vi "MPS_transmit_receive.vi"(4 "samples per readout":i32=16000, 5 "Use Bias?":bool, 9 "InputChans":enum16{"Rx", "BiasIMon", "TxIMon", "BMon"}(ring), 10 "channel input for max readouts":T1, 11 "Measurement Queue":refnum<queue>) -> ()   [LabVIEW 2021]
doc: "This VI is responsible for collecting the data of the MPI experiment from the DAQ and it writes the data of the output waveforms to the DAQ. Generally, this VI can be operated in two modes: Continuous or non-continuous mode. In non-continuous mode, a finite number of samples is read from the ADC and a finite number of samples is written to the DAC. After playing these waveforms and acquiring the samples, the VI stops. The number of samples is determined by the product of \"samples per readout\" and the \"max readouts\" number passed to the VI via a channel structure. The latter allows to update the stopping condition while the acquisition is already running. Acquired data is written to a queue (has to be provided as an input) from which the main VI can then dequeue the readout buckets. Therefore, the sub-VI can be seen as the producer loop while the consumer loop is located in the main VI.\nIn continuous mode, a finite waveform sample is repeated over and over until the data acquisition reaches the set limit or it is stopped. \nInternally, the VI has three different DAQ tasks: Analog input acquisition, analog output generation and digital input acquisition. The analog input acquisition task is the \"master task\" and all other tasks are triggered when the analog data acquisition starts. \nMost of the DAQ settings are read from the global variables (including channel, channel type and sampling rate).\nThe rotary position is taken in the middle of the readout bucket. \nFor safety reasons, the VI ensures that zeros are written to the DAQ when stopping the VI properly."
uses:
  <extravilib>/ChannelInstances/Tag-dbl/))Channel.ctl
  <vilib>/DAQmx/write.llb/DAQmx Write (Analog 1D Wfm NChan NSamp).vi
  <vilib>/DAQmx/read.llb/DAQmx Read (Analog Wfm 1Chan NSamp).vi
  MPS_global_variables.vi
  <vilib>/DAQmx/create/channels.llb/DAQmx Create Channel (AI-Voltage-Basic).vi
  <vilib>/DAQmx/configure/timing.llb/DAQmx Timing (Sample Clock).vi
  <vilib>/DAQmx/configure/trigger.llb/DAQmx Start Trigger (None).vi
  <vilib>/Waveform/WDTOps.llb/WDT Number of Waveform Samples DBL.vi
  <vilib>/DAQmx/create/channels.llb/DAQmx Create Channel (AO-Voltage-Basic).vi
  <vilib>/DAQmx/configure/trigger.llb/DAQmx Start Trigger (Digital Edge).vi
  <vilib>/DAQmx/miscellaneous.llb/DAQmx Fill In Error Info.vi
  <extravilib>/ChannelInstances/Tag-dbl/EndpointRead.vi
  <extravilib>/ChannelInstances/Tag-dbl.lvlib
  <resource>/objmgr/daqmx.rc
  <vilib>/measure/NI_MABase.lvlib
panel:
  out "output cluster":cluster{"Fs":dbl, "#s":dbl}
  out "Input waveforms 2":dbl[](graph)
  out "sample rate":dbl
  out "Sample rate actual":dbl
  out "number of samples written per channel":u32
  out "AI while loop i":i32
  out "AO while loop i":i32
  out "element":dbl
  out "Input waveforms":dynamicdata(graph)=[{"t0"=timestamp(5.936 s since 1904-01-01), "dt"=1e-06, "Y"=array[16000 elements]}, {"t0"=timestamp(5.936 s since 1904-01-01), "dt"=1e-06, "Y"=array[16000 elements]}]
  out "Transmit stopped":bool=TRUE
  out "current readout no":i32
  out "RX":waveform(dbl)(graph)
  out "Data aquisition stopped":bool=TRUE
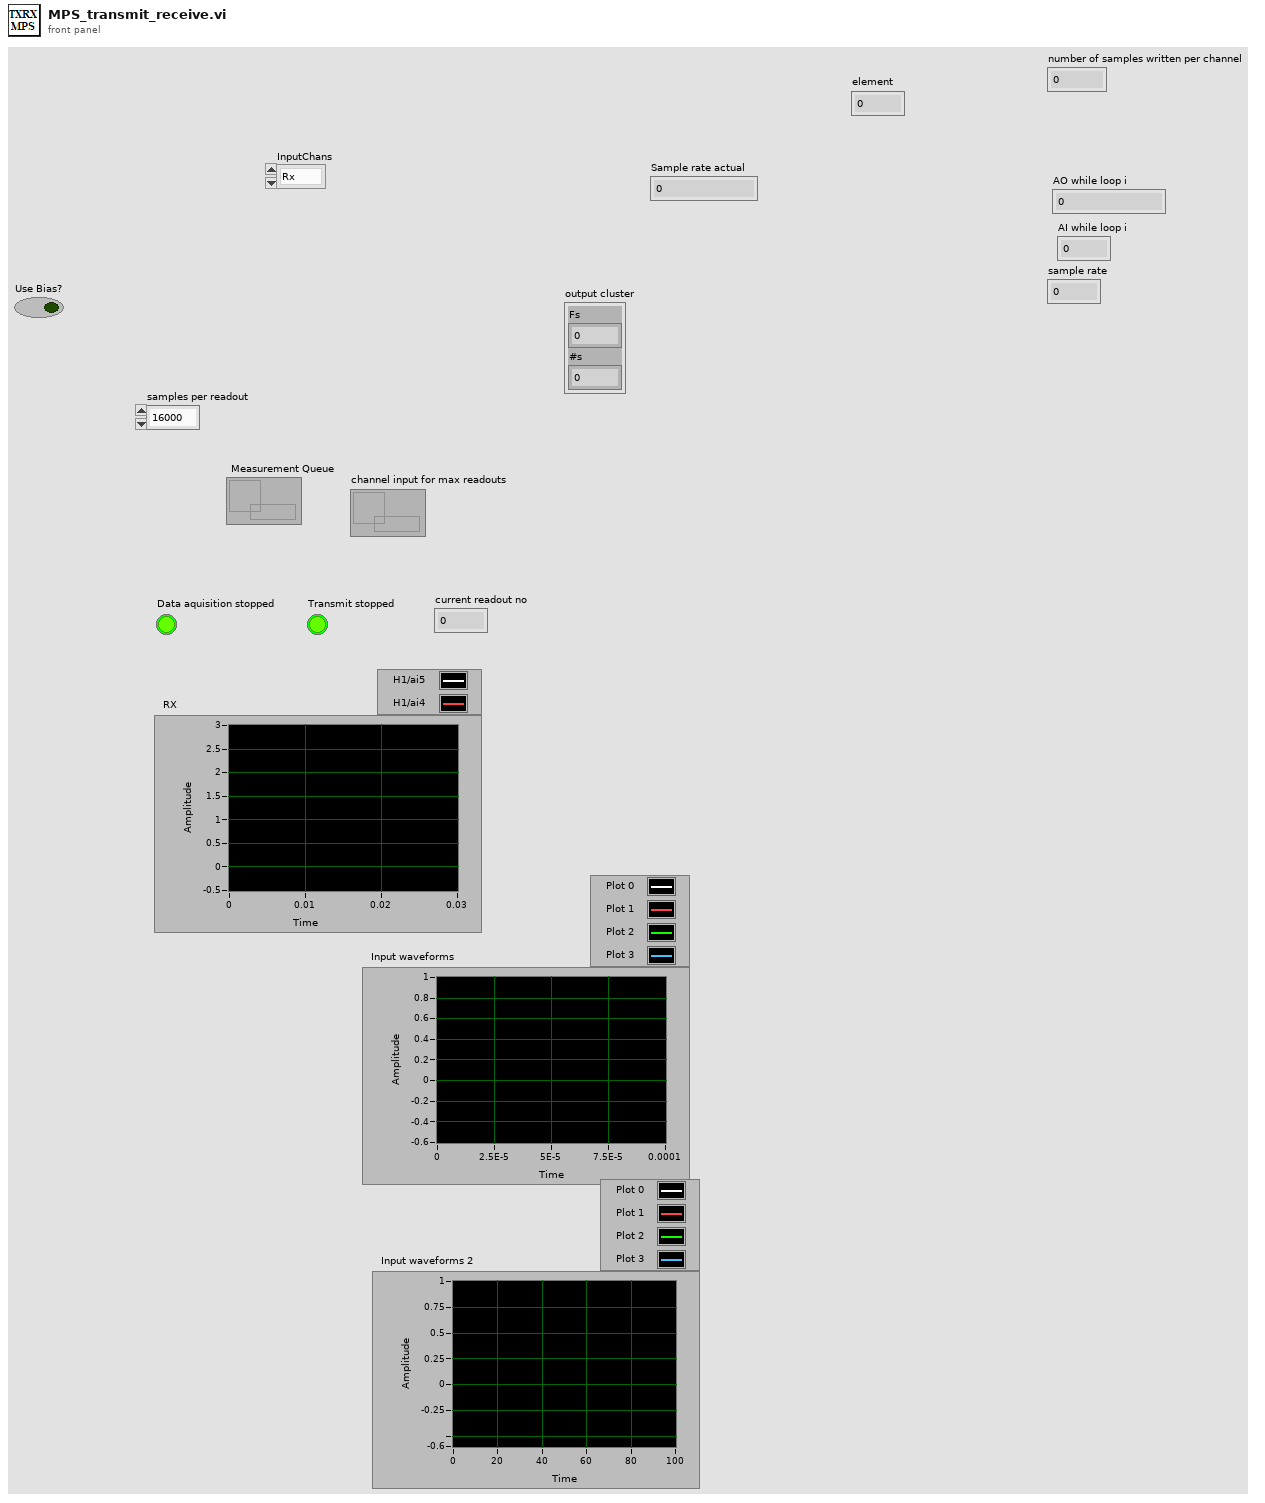
[diagram p1: front panel]
types:
  T1 = typedef "Tag-dbl.lvlib/))Channel.ctl" = refnum<queue>
  T2 = cluster{"sample rate":dbl, "Tx freq":dbl, "Tx amp":dbl, "Tx cycles\nSpectroscopy":dbl, "Bias amp":dbl, "Bias freq":dbl, "Receive range":dbl, "Bias Periods\nMagnetometry":dbl, "Tx Freq Division Factor":dbl, "Drive Periods per Bias":dbl, "TX harmonics":dbl[]}
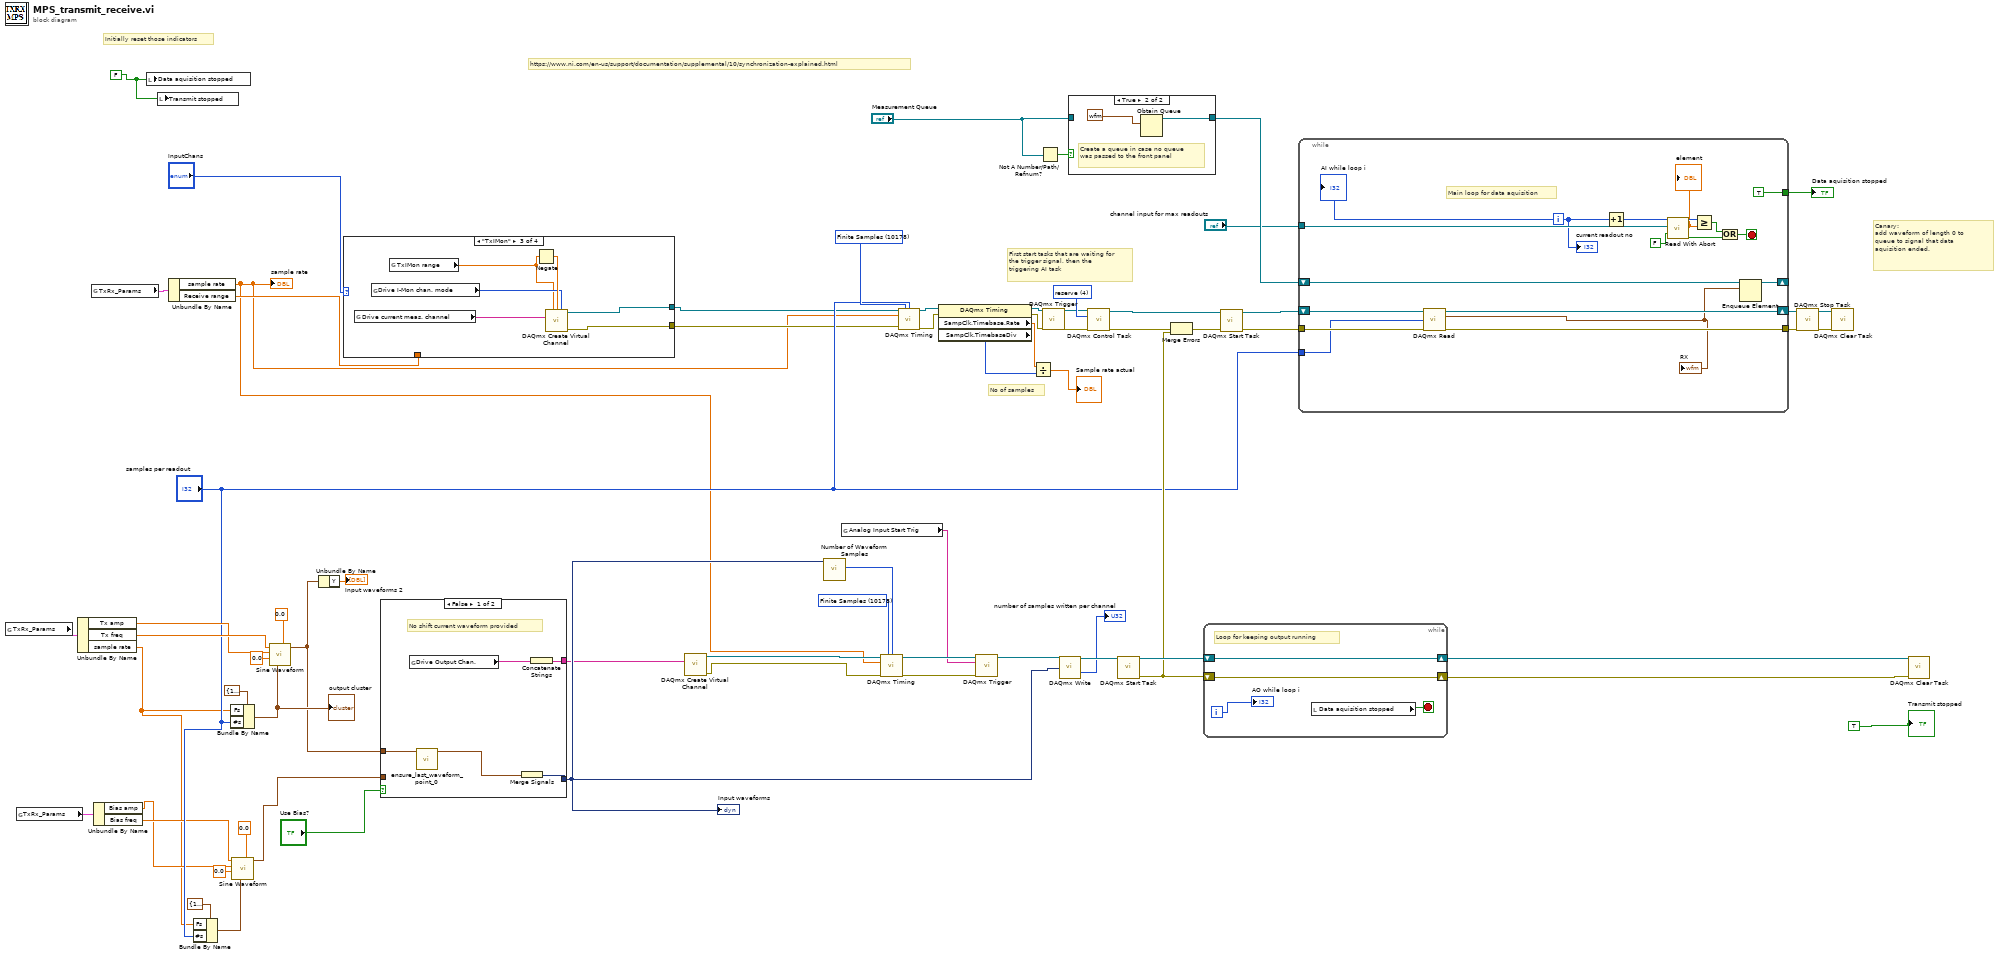
[diagram p0: block diagram]
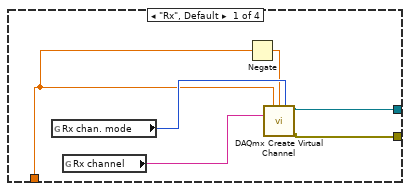
[diagram p2: hidden frame]
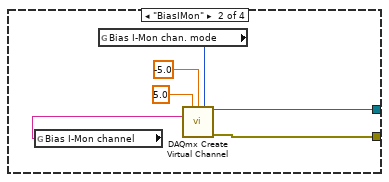
[diagram p3: hidden frame]
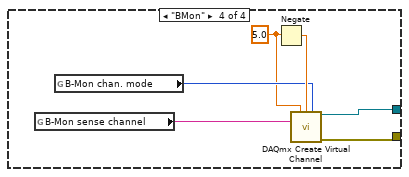
[diagram p4: hidden frame]
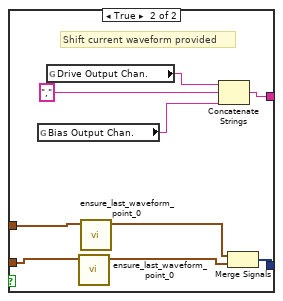
[diagram p6: hidden frame]
diagram:
  w47 = 10178 items=["Finite Samples"=10178, "Continuous Samples"=10123, "Hardware Timed Single Point"=12522] ("sample mode")
  w56 = 4 items=["verify"=2, "reserve"=4, "commit"=3, "unreserve"=5, "abort"=6] ("action")
  w31 = 10178 items=["Finite Samples"=10178, "Continuous Samples"=10123, "Hardware Timed Single Point"=12522] ("sample mode")
  w52 = FALSE ("Data aquisition stopped 2")
  # "https://www.ni.com/en-us/support/documentation/supplemental/10/synchronization-explained.html"
  # "First start tasks that are waiting for the trigger signal, then the triggering AI task"
  # "Initially reset those indicators"
  # "Canary:\nadd waveform of length 0 to queue to signal that data aquisition ended."
  # "No of samples"
  n1 = global read "MPS_global_variables.vi" "TxRx_Params"() -> (w27:T2)
  n2 = global read "MPS_global_variables.vi" "TxRx_Params"() -> (w26:T2)
  n3 = Unbundle By Name(w27) -> ("Tx amp"=w19:dbl, "Tx freq"=w20:dbl, "sample rate"=w11:dbl)
  n4 = global read "MPS_global_variables.vi" "TxRx_Params"() -> (w33:T2)
  n5 = Unbundle By Name(w26) -> ("Bias amp"=w12:dbl, "Bias freq"=w13:dbl)
  n6 = local write "Data aquisition stopped"(w52) -> ()
  n7 = local write "Transmit stopped"(w52) -> ()
  n8 = Unbundle By Name(w33) -> ("sample rate"=w1:dbl, "Receive range"=w5:dbl)
  "sample rate" <- w1
  n9 = Bundle By Name(cluster=cluster{"Fs":dbl, "#s":dbl} {"Fs"=1000.0, "#s"=1000.0} ("sampling info"), "Fs"=w11, "#s"="samples per readout") -> (w18:cluster{"Fs":dbl, "#s":dbl})
  n10 = Bundle By Name(cluster=cluster{"Fs":dbl, "#s":dbl} {"Fs"=1000.0, "#s"=1000.0} ("sampling info"), "Fs"=w11, "#s"="samples per readout") -> (w21:cluster{"Fs":dbl, "#s":dbl})
  "output cluster" <- w21
  n11 = call <vilib>:"Sine Waveform.vi"("offset"=0.0, "sampling info"=w18, "phase"=0.0, "amplitude"=w12, "frequency"=w13) -> ("signal out"=w14:waveform(dbl))  [unwired: 5 in, 1 out]
  n12 = call <vilib>:"Sine Waveform.vi"("offset"=0.0, "sampling info"=w21, "phase"=0.0, "amplitude"=w19, "frequency"=w20) -> ("signal out"=w8:waveform(dbl))  [unwired: 5 in, 1 out]
  n13 = Unbundle By Name(w8) -> ("Y"=→"Input waveforms 2":dbl[])
  n14 = case shown="\"TxIMon\"" "InputChans" {
    tunnel: w5 -> [w72 _ _ _]
    tunnel: [w71 w77 w84 w89] -> w4
    tunnel: [w70 w76 w83 w88] -> w3
    frame "Rx", Default {
      n15 = global read "MPS_global_variables.vi" "Rx chan. mode"() -> (w74:i32)
      n16 = global read "MPS_global_variables.vi" "Rx channel"() -> (w75:tag)
      n17 = Negate(x=w72) -> (-x=w73:dbl)
      n18 = call-poly <vilib>:"DAQmx Create Virtual Channel.vi"("maximum value"=w72, "minimum value"=w73, "input terminal configuration"=w74, "physical channels"=w75) -> ("task out"=w71:refnum<k21>, "error out"=w70:errorcluster)  [unwired: 10 in]
    }
    frame "BiasIMon" {
      n19 = global read "MPS_global_variables.vi" "Bias I-Mon channel"() -> (w79:tag)
      n20 = global read "MPS_global_variables.vi" "Bias I-Mon chan. mode"() -> (w78:i32)
      n21 = call-poly <vilib>:"DAQmx Create Virtual Channel.vi"("maximum value"=5.0, "minimum value"=-5.0, "input terminal configuration"=w78, "physical channels"=w79) -> ("task out"=w77:refnum<k21>, "error out"=w76:errorcluster)  [unwired: 10 in]
    }
    frame "TxIMon" {
      n22 = global read "MPS_global_variables.vi" "Drive current meas. channel"() -> (w86:tag)
      n23 = global read "MPS_global_variables.vi" "Drive I-Mon chan. mode"() -> (w85:i32)
      n24 = global read "MPS_global_variables.vi" "TxIMon range"() -> (w82:dbl)
      n25 = Negate(x=w82) -> (-x=w87:dbl)
      n26 = call-poly <vilib>:"DAQmx Create Virtual Channel.vi"("maximum value"=w82, "minimum value"=w87, "input terminal configuration"=w85, "physical channels"=w86) -> ("task out"=w84:refnum<k21>, "error out"=w83:errorcluster)  [unwired: 10 in]
    }
    frame "BMon" {
      w90 = 5.0 ("Receive range")
      n27 = global read "MPS_global_variables.vi" "B-Mon sense channel"() -> (w92:tag)
      n28 = global read "MPS_global_variables.vi" "B-Mon chan. mode"() -> (w91:i32)
      n29 = Negate(x=w90) -> (-x=w93:dbl)
      n30 = call-poly <vilib>:"DAQmx Create Virtual Channel.vi"("maximum value"=w90, "minimum value"=w93, "input terminal configuration"=w91, "physical channels"=w92) -> ("task out"=w89:refnum<k21>, "error out"=w88:errorcluster)  [unwired: 10 in]
    }
  }
  n31 = case shown="False" "Use Bias?" {
    tunnel: [w96 w107] -> w32
    tunnel: w14 -> [_ w104]
    tunnel: w8 -> [w97 w101]
    tunnel: [w98 w106] -> w59
    frame False {
      # "No shift current waveform provided"
      n32 = global read "MPS_global_variables.vi" "Drive Output Chan."() -> (w94:tag)
      n33 = call "ensure_last_waveform_point_0.vi"("Waveform in"=w97) -> ("Waveform out"=w95:waveform(dbl))  [unwired: 10 in]
      n34 = Merge Signals(w95) -> (w98:dynamicdata)
      n35 = Concatenate Strings(w94) -> (w96:string)
    }
    frame True {
      # "Shift current waveform provided"
      n36 = global read "MPS_global_variables.vi" "Bias Output Chan."() -> (w100:tag)
      n37 = global read "MPS_global_variables.vi" "Drive Output Chan."() -> (w99:tag)
      n38 = call "ensure_last_waveform_point_0.vi"("Waveform in"=w104) -> ("Waveform out"=w103:waveform(dbl))  [unwired: 10 in]
      n39 = call "ensure_last_waveform_point_0.vi"("Waveform in"=w101) -> ("Waveform out"=w102:waveform(dbl))  [unwired: 10 in]
      n40 = Concatenate Strings(w99, "," ("string"), w100) -> (w107:string)
      n41 = Merge Signals(w102, w103) -> (w106:dynamicdata)
    }
  }
  "Input waveforms" <- w59
  n42 = call-poly <vilib>:"DAQmx Create Virtual Channel.vi"("physical channels"=w32) -> ("task out"=w35:refnum<k21>, "error out"=w34:errorcluster)  [unwired: 13 in]
  n43 = call-poly <vilib>:"Number of Waveform Samples.vi"("waveform in"=w59) -> ("number of samples"=w58:i32)  [unwired: 8 in, 2 out]
  n44 = global read "MPS_global_variables.vi" "Analog Input Start Trig"() -> (w30:tag)
  n45 = call-poly <vilib>:"DAQmx Timing.vi"("task/channels in"=w35, "sample mode"=w31, "samples per channel"=w58, "rate"=w1, "error in"=w34) -> ("task out"=w69:refnum<k21>, "error out"=w68:errorcluster)  [unwired: 9 in]
  n46 = call-poly <vilib>:"DAQmx Timing.vi"("task/channels in"=w4, "sample mode"=w47, "samples per channel"="samples per readout", "rate"=w1, "error in"=w3) -> ("task out"=w42:refnum<k21>, "error out"=w41:errorcluster)  [unwired: 9 in]
  n47 = property class="DAQmx Timing"(reference=w42, error in=w41) -> (reference out=w39:refnum<k21>, error out=w40:errorcluster, "SampClk.Timebase.Rate"=w38:dbl, "SampClk.TimebaseDiv"=w37:u32)
  n48 = call-poly <vilib>:"DAQmx Trigger.vi"("task/channels in"=w69, "source"=w30, "error in"=w68) -> ("task out"=w67:refnum<k21>)  [unwired: 11 in, 1 out]
  n49 = Divide(x=w38, y=w37) -> (x/y=→"Sample rate actual":dbl)
  n50 = Not A Number/Path/Refnum?(number/path/refnum="Measurement Queue") -> (NaN/Path/Refnum?=w65:bool)
  n51 = call-poly <vilib>:"DAQmx Trigger.vi"("task/channels in"=w39, "error in"=w40) -> ("task out"=w54:refnum<k21>, "error out"=w55:errorcluster)  [unwired: 12 in]
  n52 = call-poly <vilib>:"DAQmx Write.vi"("task/channels in"=w67, "data"=w59) -> ("task out"=w60:refnum<k21>, "number of samples written per channel"=→"number of samples written per channel":u32)  [unwired: 11 in, 1 out]
  n53 = case shown="True" w65 {
    tunnel: "Measurement Queue" -> [w108 _]
    tunnel: [w108 w109] -> w64
    frame False {
    }
    frame True {
      # "Create a queue in case no queue was passed to the front panel"
      n54 = Obtain Queue(element data type=waveform(dbl) {"t0"=timestamp(0 s since 1904-01-01), "dt"=1.0, "Y"=[]} ("Waveform")) -> (queue out=w109:refnum<queue>)  [unwired: 4 in, 2 out]
    }
  }
  n55 = call <vilib>:"DAQmx Control Task.vi"("task/channels in"=w54, "action"=w56, "error in"=w55) -> ("task out"=w46:refnum<k21>, "error out"=w53:errorcluster)  [unwired: 11 in]
  n56 = call <vilib>:"DAQmx Start Task.vi"("task/channels in"=w60) -> ("task out"=w57:refnum<k21>, "error out"=w28:errorcluster)  [unwired: 13 in]
  n57 = Merge Errors(w53, w28) -> (w29:errorcluster)
  n58 = while {
    shift-right: [w112] -> w61
    shift-left: w57 -> [w112]
    shift-right: [w113] -> w62
    shift-left: w28 -> [w113]
    i -> [w111]
    stop <- w114 stop-if-true
    # "Loop for keeping output running"
    n59 = local read "Data aquisition stopped"() -> (w114:bool)
    "AO while loop i" <- w111
  }
  n60 = call <vilib>:"DAQmx Start Task.vi"("task/channels in"=w46, "error in"=w29) -> ("task out"=w45:refnum<k21>, "error out"=w44:errorcluster)  [unwired: 12 in]
  n61 = while {
    tunnel: w44 -> [w118]
    tunnel: "samples per readout" -> [w116]
    shift-right: [w128] -> _
    shift-left: w64 -> [w129]
    tunnel: [TRUE] -> w66
    tunnel: "channel input for max readouts" -> [w127]
    shift-right: [w119] -> w49
    shift-left: w45 -> [w131]
    tunnel: [w117] -> w48
    i -> [w125]
    stop <- w120 stop-if-true
    # "Main loop for data aquisition"
    n62 = call-poly <vilib>:"DAQmx Read.vi"("task/channels in"=w131, "number of samples per channel"=w116, "error in"=w118) -> ("task out"=w119:refnum<k21>, "data"=w115:waveform(dbl), "error out"=w117:errorcluster)  [unwired: 10 in]
    "RX" <- w115
    n63 = Increment(x=w125) -> (x+1=w124:i32)
    n64 = call <extravilib>:"Read With Abort.vi"("abort"=FALSE, "channel"=w127) -> ("element"=w123:dbl, "aborted?"=w121:bool)  [unwired: 7 in, 1 out]
    "element" <- w123
    n65 = Greater Or Equal?(x=w124, y=w123) -> (x >= y?=w122:bool)
    n66 = Or(x=w122, y=w121) -> (x .or. y?=w120:bool)
    n67 = Enqueue Element(queue=w129, element=w115) -> (queue out=w128:refnum<queue>)  [unwired: 2 in, 2 out]
    "current readout no" <- w125
    "AI while loop i" <- w125
  }
  "Data aquisition stopped" <- w66
  n68 = call <vilib>:"DAQmx Stop Task.vi"("task/channels in"=w49, "error in"=w48) -> ("task out"=w51:refnum<k21>, "error out"=w50:errorcluster)  [unwired: 12 in]
  n69 = call <vilib>:"DAQmx Clear Task.vi"("task in"=w51, "error in"=w50) -> ()  [unwired: 13 in, 1 out]
  n70 = call <vilib>:"DAQmx Clear Task.vi"("task in"=w61, "error in"=w62) -> ()  [unwired: 13 in, 1 out]
  "Transmit stopped" <- TRUE
